vi "ConvertToDataString.vi"(8 "error in":errorcluster, 9 "Data":string[][](array[string]), 10 "DataName":string[](array[string])) -> (0 "error out":errorcluster, 2 "DataString":string)   [LabVIEW 2015]
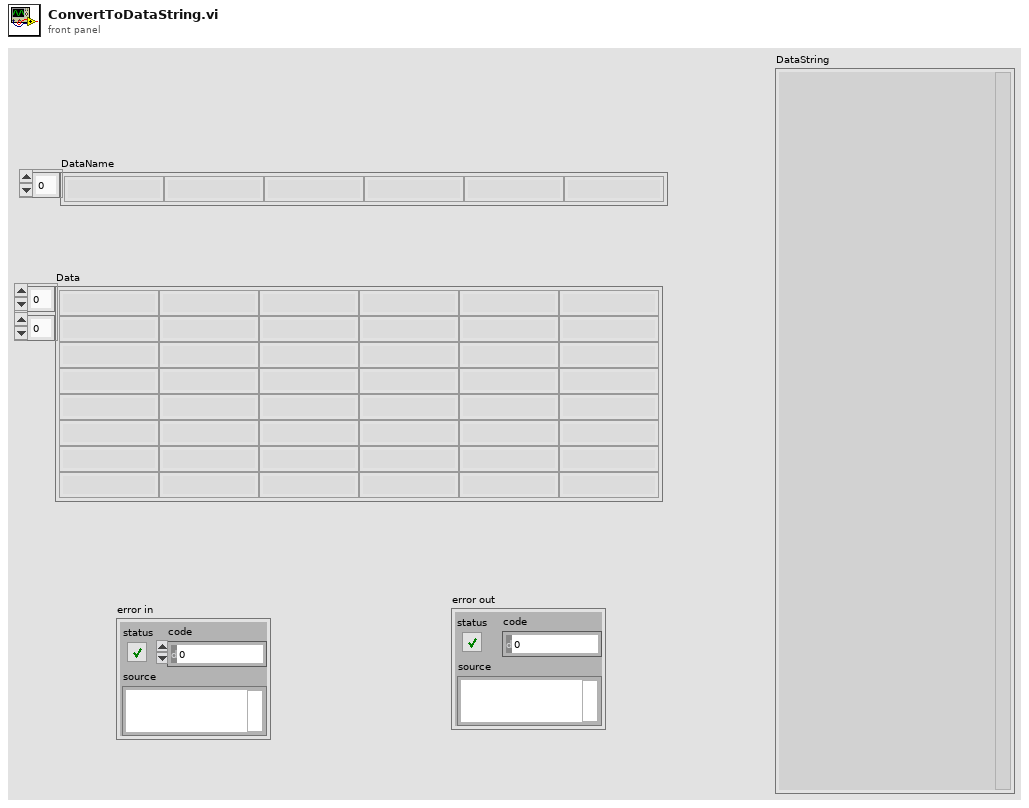
[diagram p1: front panel]
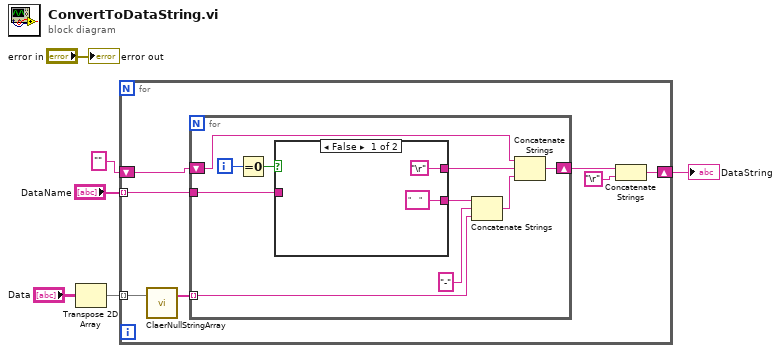
[diagram p0: block diagram]
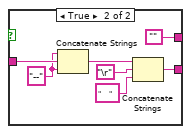
[diagram p2: hidden frame]
diagram:
  n1 = Transpose 2D Array(2D array="Data") -> (transposed array=w2:string[][])
  n2 = for {
    tunnel: "DataName" -> [w13] mode=indexing
    tunnel: w2 -> [w12] mode=indexing
    shift-right: [w7] -> w6
    shift-left: "" -> [w10]
    n3 = call <userlib>:"ClaerNullStringArray.vi"("Array in"=w12) -> ("Array out"=w11:string[])  [unwired: 18 in]
    n4 = for {
      tunnel: w11 -> [w22] mode=indexing
      tunnel: w13 -> [w15]
      shift-right: [w19] -> w8
      shift-left: w10 -> [w20]
      i -> [w21]
      n5 = Equal To 0?(x=w21) -> (x = 0?=w17:bool)
      n6 = case shown="False" w17 {
        tunnel: ["    " w31] -> w16
        tunnel: w15 -> [_ w28]
        tunnel: ["\r" ""] -> w14
        frame False {
        }
        frame True {
          w27 = "--"
          n7 = Concatenate Strings(w27, w28, w27) -> (w29:string)
          n8 = Concatenate Strings(w29, "\r", "    ") -> (w31:string)
        }
      }
      n9 = Concatenate Strings(w16, "-" ("string"), w22) -> (w18:string)
      n10 = Concatenate Strings(w20, w14, w18) -> (w19:string)
    }
    n11 = Concatenate Strings(w8, "\r") -> (w7:string)
  }
  "DataString" <- w6
  "error out" <- "error in"
